vi "prompt_user_for_number_input.vi"() -> (0 "Power Reading out":dbl)   [LabVIEW 2019]
panel:
  in  "OK Button":bool
  in  "Power Reading (uW)":dbl
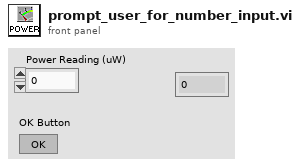
[diagram p1: front panel]
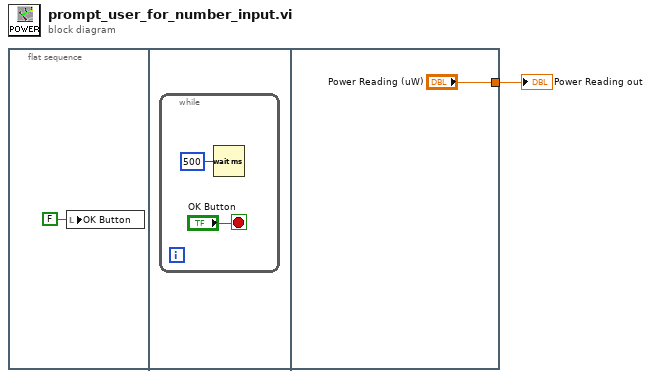
[diagram p0: block diagram]
diagram:
  n1 = flat-sequence {
    tunnel: ["Power Reading (uW)"] -> w1
    frame #0 {
      n2 = local write "OK Button"(FALSE ("OK Button")) -> ()
    }
    frame #1 {
      n3 = while {
        stop <- "OK Button" stop-if-true
        n4 = Wait (ms)(milliseconds to wait=u32 500) -> ()  [unwired: 1 out]
      }
    }
    frame #2 {
    }
  }
  "Power Reading out" <- w1
